vi "ex_BTD.vi"() -> ()   [LabVIEW 2022 SP3]
doc: "This is the VI which is a simple Blood Test Device"
uses:
  #typedef_Blood_Testing_Device_Task.ctl
  #typedef_Kind_Of_Operation_BTD.ctl
  #typedef_Blood_Testing_Device_States.ctl
  #typedef_TimerAction.ctl
  #typed_BTD_ProgramData.ctl
panel:
  out "Centrifugation (slide)":bool
  out "Kind Of Opeartion":T1
  in  "Lid Open":bool
  in  "Centrifugation":bool
  in  "Start":bool
  in  "Dial":T2 scale=0.0..4.0
  in  "stop":bool
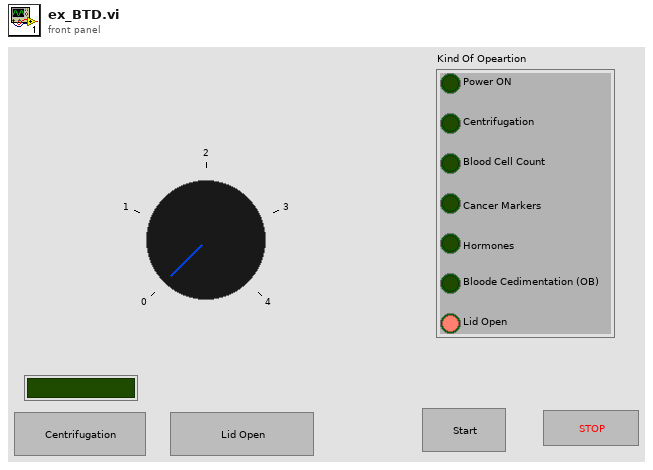
[diagram p1: front panel]
types:
  T1 = typedef "#typedef_Kind_Of_Operation_BTD.ctl" = cluster{"Power ON":bool, "Centrifugation":bool, "Blood Cell Count":bool, "Cancer Markers":bool, "Hormones":bool, "Bloode Cedimentation (OB)":bool, "Lid Open":bool}
  T2 = typedef "#typedef_Blood_Testing_Device_Task.ctl" = i32
  T3 = typedef "#typedef_Blood_Testing_Device_States.ctl" = enum16{"Blood Cedimentation (OB)", "Hormones", "Cancer Markers", "Blood Cell Count", "Centrifugation", "Initialization", "Exit", "Error Handler", "Centrifugation Led On", "Wait For Event"}
  T4 = typedef "#typedef_TimerAction.ctl" = enum16{"Reset", "TimeElapsed"}
  T5 = typedef "#typed_BTD_ProgramData.ctl" = cluster{"Kind Of Opearion":T1, "Task":T2}
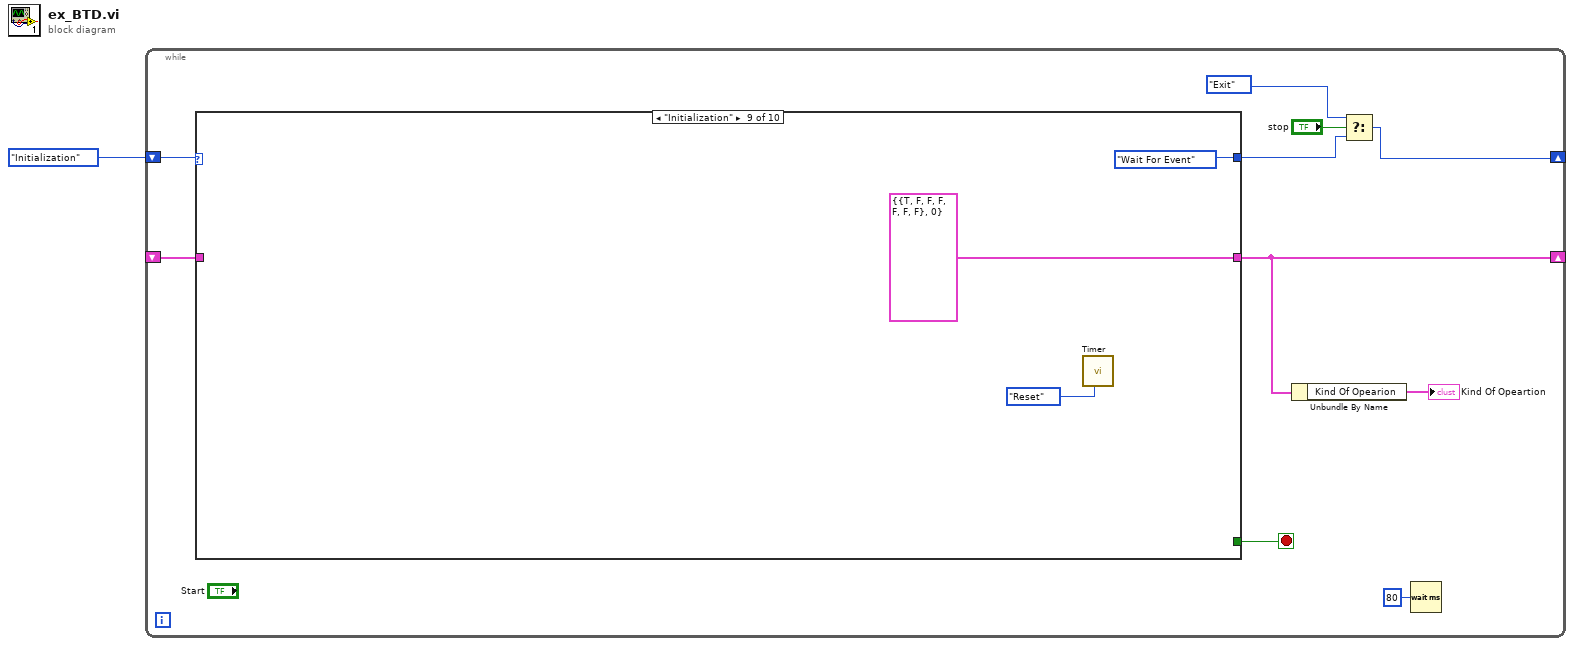
[diagram p0: block diagram]
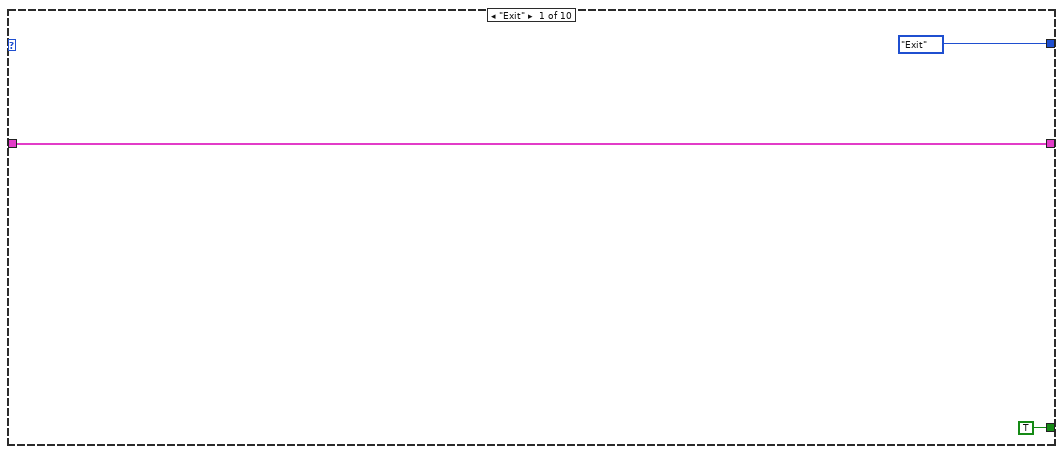
[diagram p2: hidden frame]
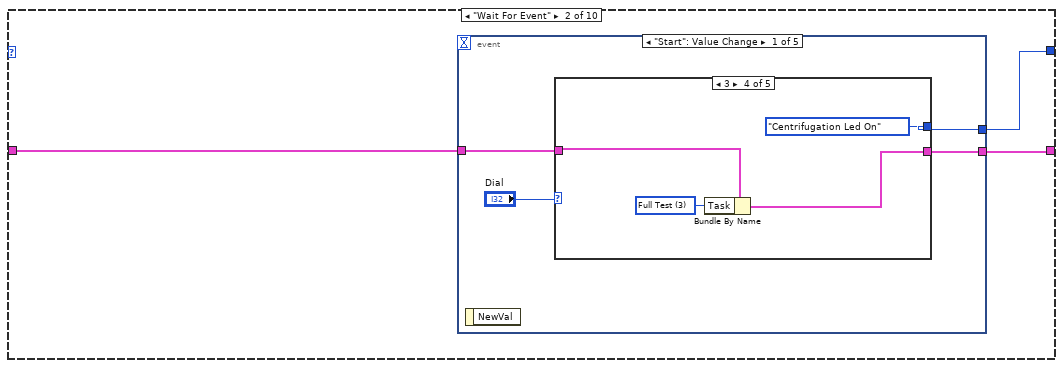
[diagram p3: hidden frame]
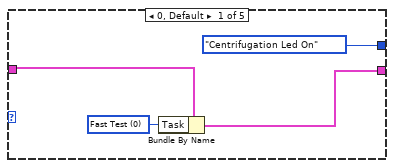
[diagram p4: hidden frame]
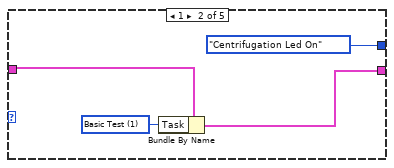
[diagram p5: hidden frame]
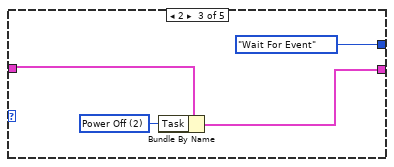
[diagram p6: hidden frame]
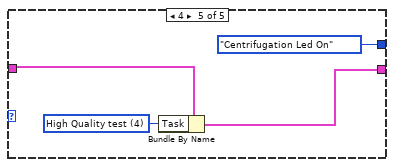
[diagram p7: hidden frame]
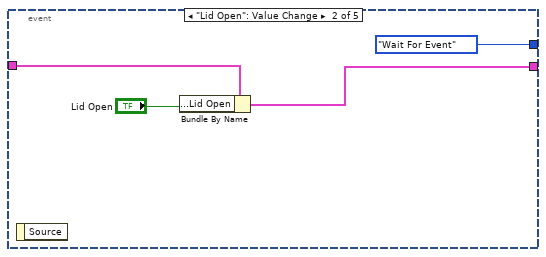
[diagram p8: hidden frame]
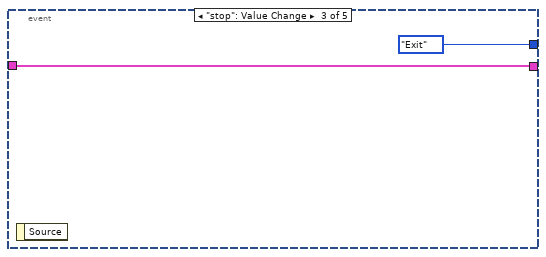
[diagram p9: hidden frame]
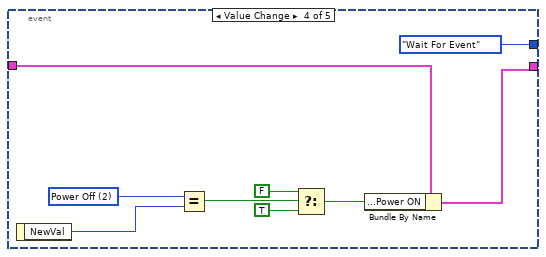
[diagram p10: hidden frame]
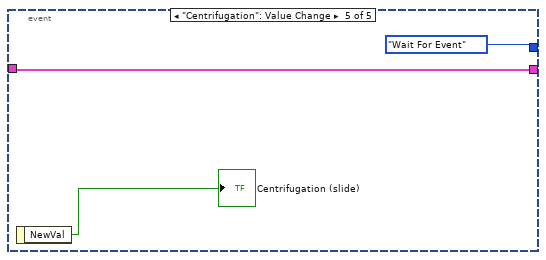
[diagram p11: hidden frame]
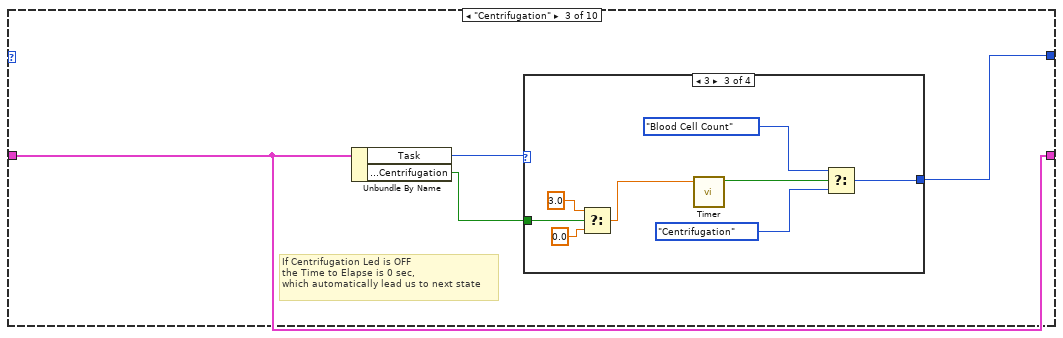
[diagram p12: hidden frame]
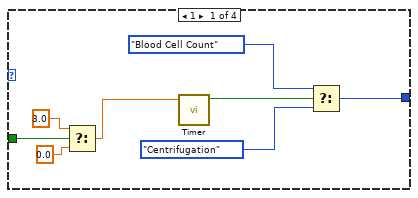
[diagram p13: hidden frame]
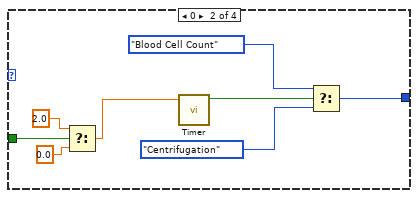
[diagram p14: hidden frame]
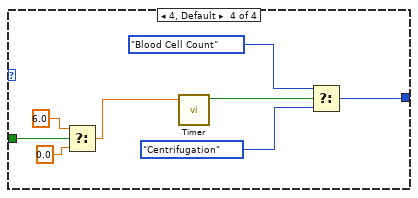
[diagram p15: hidden frame]
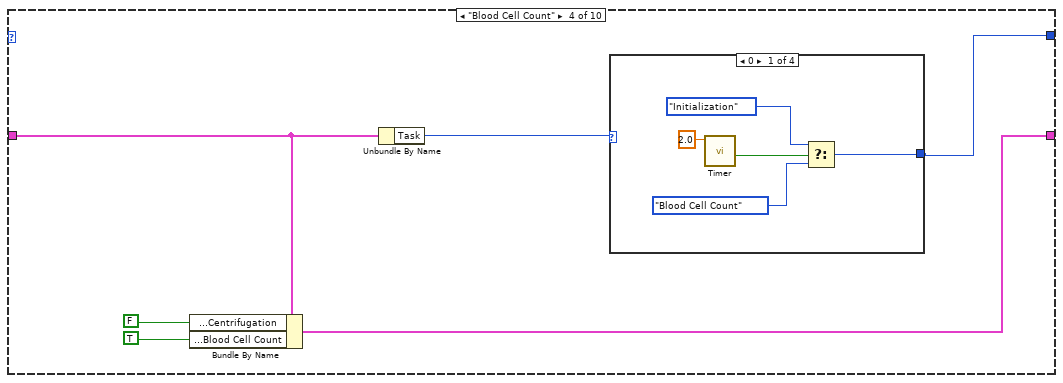
[diagram p16: hidden frame]
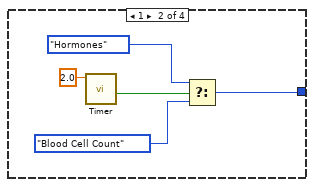
[diagram p17: hidden frame]
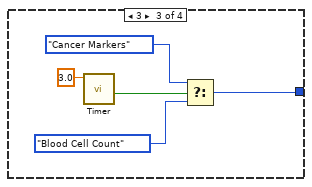
[diagram p18: hidden frame]
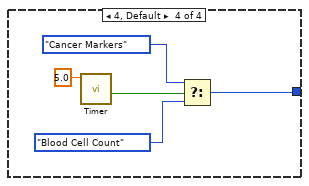
[diagram p19: hidden frame]
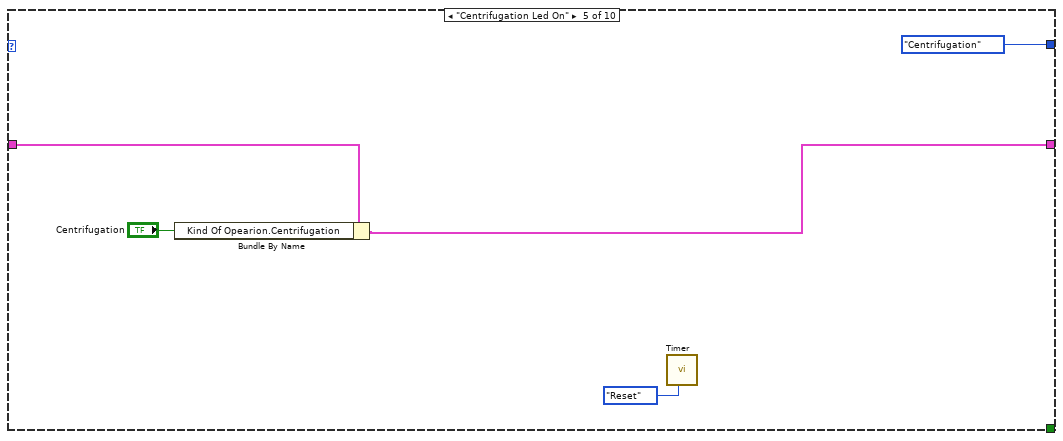
[diagram p20: hidden frame]
diagram:
  n1 = while {
    shift-right: [w4] -> _
    shift-left: #typedef_Blood_Testing_Device_States."Initialization" ("SM_States") -> [w11]
    shift-right: [w3] -> _
    shift-left: _ -> [w10]
    stop <- w9 stop-if-true
    n2 = case shown="\"Initialization\"" w11 {
      tunnel: [w13 w16 w60 w98 w124 w129 w146 w167 T5 {"Kind Of Opearion"={"Power ON"=TRUE, "Centrifugation"=FALSE, "Blood Cell Count"=FALSE, "Cancer Markers"=FALSE, "Hormones"=FALSE, "Bloode Cedimentation (OB)"=FALSE, "Lid Open"=FALSE}, "Task"=0} ("BTD_ProgramData") w190] -> w3
      tunnel: [#typedef_Blood_Testing_Device_States."Exit" ("SM_States") w15 w62 w97 #typedef_Blood_Testing_Device_States."Centrifugation" ("SM_States") w128 w145 w166 #typedef_Blood_Testing_Device_States."Wait For Event" ("SM_States") #typedef_Blood_Testing_Device_States."Exit" ("SM_States")] -> w7
      tunnel: w10 -> [w13 w17 w60 w100 w126 w131 w148 w169 _ w190]
      tunnel: [TRUE _ _ _ _ _ _ _ _ w189] -> w9
      frame "Exit" {
      }
      frame "Wait For Event" {
        n3 = event shown="[0] \"Start\": Value Change" {
          selector: _ -> [_ _ _ _ _]
          dyn-events: _ -> [_ _ _ _ _]
          timeout: _ -> [_ _ _ _ _]
          tunnel: w17 -> [w20 w45 w47 w50 w57]
          tunnel: [w19 w43 w47 w49 w57] -> w16
          tunnel: [w18 #typedef_Blood_Testing_Device_States."Wait For Event" ("SM_States") #typedef_Blood_Testing_Device_States."Exit" ("SM_States") #typedef_Blood_Testing_Device_States."Wait For Event" ("SM_States") #typedef_Blood_Testing_Device_States."Wait For Event" ("SM_States")] -> w15
          event "Start": Value Change {
            n4 = event-data() -> ()  [unwired: 1 in, 1 out]
            n5 = case shown="3" "Dial" {
              tunnel: w20 -> [w25 w29 w33 w37 w41]
              tunnel: [w23 w27 w31 w35 w39] -> w19
              tunnel: [#typedef_Blood_Testing_Device_States."Centrifugation Led On" ("SM_States") #typedef_Blood_Testing_Device_States."Centrifugation Led On" ("SM_States") #typedef_Blood_Testing_Device_States."Wait For Event" ("SM_States") #typedef_Blood_Testing_Device_States."Centrifugation Led On" ("SM_States") #typedef_Blood_Testing_Device_States."Centrifugation Led On" ("SM_States")] -> w18
              frame 0, Default {
                w24 = T2 0 items=["Fast Test", "Basic Test", "Power Off", "Full Test", "High Quality test"] ("Task")
                n6 = Bundle By Name(cluster=w25, "Task"=w24) -> (w23:T5)
              }
              frame 1 {
                w28 = T2 1 items=["Fast Test", "Basic Test", "Power Off", "Full Test", "High Quality test"] ("Task")
                n7 = Bundle By Name(cluster=w29, "Task"=w28) -> (w27:T5)
              }
              frame 2 {
                w32 = T2 2 items=["Fast Test", "Basic Test", "Power Off", "Full Test", "High Quality test"] ("Task")
                n8 = Bundle By Name(cluster=w33, "Task"=w32) -> (w31:T5)
              }
              frame 3 {
                w36 = T2 3 items=["Fast Test", "Basic Test", "Power Off", "Full Test", "High Quality test"] ("Task")
                n9 = Bundle By Name(cluster=w37, "Task"=w36) -> (w35:T5)
              }
              frame 4 {
                w40 = T2 4 items=["Fast Test", "Basic Test", "Power Off", "Full Test", "High Quality test"] ("Task")
                n10 = Bundle By Name(cluster=w41, "Task"=w40) -> (w39:T5)
              }
            }
          }
          event "Lid Open": Value Change {
            n11 = event-data() -> ()  [unwired: 1 in, 1 out]
            n12 = Bundle By Name(cluster=w45, "Kind Of Opearion.Lid Open"="Lid Open") -> (w43:T5)
          }
          event "stop": Value Change {
            n13 = event-data() -> ()  [unwired: 1 in, 1 out]
          }
          event Value Change {
            w52 = T2 2 items=["Fast Test", "Basic Test", "Power Off", "Full Test", "High Quality test"] ("x")
            n14 = event-data() -> ("NewVal"=w56:T2)  [unwired: 1 in]
            n15 = Equal?(x=w52, y=w56) -> (x = y?=w55:bool)
            n16 = Select(t=FALSE, s=w55, f=TRUE) -> (s? t:f=w51:bool)
            n17 = Bundle By Name(cluster=w50, "Kind Of Opearion.Power ON"=w51) -> (w49:T5)
          }
          event "Centrifugation": Value Change {
            n18 = event-data() -> ("NewVal"=→"Centrifugation (slide)":bool)  [unwired: 1 in]
          }
        }
      }
      frame "Centrifugation" {
        # "If Centrifugation Led is OFF\nthe Time to Elapse is 0 sec,\nwhich automatically lead us to next state"
        n19 = Unbundle By Name(w60) -> ("Task"=w63:T2, "Kind Of Opearion.Centrifugation"=w61:bool)
        n20 = case shown="3" w63 {
          tunnel: [w68 w76 w84 w92] -> w62
          tunnel: w61 -> [w67 w75 w83 w91]
          frame 1 {
            n21 = Select(t=3.0, s=w67, f=0.0) -> (s? t:f=w64:dbl)
            n22 = call "Timer.vi"("Time To Elapse"=w64) -> ("Time Elapsed?"=w70:bool)  [unwired: 8 in, 2 out]
            n23 = Select(t=#typedef_Blood_Testing_Device_States."Blood Cell Count" ("SM_States"), s=w70, f=#typedef_Blood_Testing_Device_States."Centrifugation") -> (s? t:f=w68:T3)
          }
          frame 0 {
            n24 = Select(t=2.0, s=w75, f=0.0) -> (s? t:f=w72:dbl)
            n25 = call "Timer.vi"("Time To Elapse"=w72) -> ("Time Elapsed?"=w78:bool)  [unwired: 8 in, 2 out]
            n26 = Select(t=#typedef_Blood_Testing_Device_States."Blood Cell Count" ("SM_States"), s=w78, f=#typedef_Blood_Testing_Device_States."Centrifugation") -> (s? t:f=w76:T3)
          }
          frame 3 {
            n27 = Select(t=3.0, s=w83, f=0.0) -> (s? t:f=w80:dbl)
            n28 = call "Timer.vi"("Time To Elapse"=w80) -> ("Time Elapsed?"=w86:bool)  [unwired: 8 in, 2 out]
            n29 = Select(t=#typedef_Blood_Testing_Device_States."Blood Cell Count" ("SM_States"), s=w86, f=#typedef_Blood_Testing_Device_States."Centrifugation") -> (s? t:f=w84:T3)
          }
          frame 4, Default {
            n30 = Select(t=6.0, s=w91, f=0.0) -> (s? t:f=w88:dbl)
            n31 = call "Timer.vi"("Time To Elapse"=w88) -> ("Time Elapsed?"=w94:bool)  [unwired: 8 in, 2 out]
            n32 = Select(t=#typedef_Blood_Testing_Device_States."Blood Cell Count" ("SM_States"), s=w94, f=#typedef_Blood_Testing_Device_States."Centrifugation") -> (s? t:f=w92:T3)
          }
        }
      }
      frame "Blood Cell Count" {
        n33 = Bundle By Name(cluster=w100, "Kind Of Opearion.Centrifugation"=FALSE, "Kind Of Opearion.Blood Cell Count"=TRUE) -> (w98:T5)
        n34 = Unbundle By Name(w100) -> ("Task"=w101:T2)
        n35 = case shown="0" w101 {
          tunnel: [w102 w107 w112 w117] -> w97
          frame 0 {
            n36 = call "Timer.vi"("Time To Elapse"=2.0) -> ("Time Elapsed?"=w106:bool)  [unwired: 8 in, 2 out]
            n37 = Select(t=#typedef_Blood_Testing_Device_States."Initialization" ("SM_States"), s=w106, f=#typedef_Blood_Testing_Device_States."Blood Cell Count" ("SM_States")) -> (s? t:f=w102:T3)
          }
          frame 1 {
            n38 = call "Timer.vi"("Time To Elapse"=2.0) -> ("Time Elapsed?"=w111:bool)  [unwired: 8 in, 2 out]
            n39 = Select(t=#typedef_Blood_Testing_Device_States."Hormones" ("SM_States"), s=w111, f=#typedef_Blood_Testing_Device_States."Blood Cell Count" ("SM_States")) -> (s? t:f=w107:T3)
          }
          frame 3 {
            n40 = call "Timer.vi"("Time To Elapse"=3.0) -> ("Time Elapsed?"=w116:bool)  [unwired: 8 in, 2 out]
            n41 = Select(t=#typedef_Blood_Testing_Device_States."Cancer Markers" ("SM_States"), s=w116, f=#typedef_Blood_Testing_Device_States."Blood Cell Count" ("SM_States")) -> (s? t:f=w112:T3)
          }
          frame 4, Default {
            n42 = call "Timer.vi"("Time To Elapse"=5.0) -> ("Time Elapsed?"=w121:bool)  [unwired: 8 in, 2 out]
            n43 = Select(t=#typedef_Blood_Testing_Device_States."Cancer Markers" ("SM_States"), s=w121, f=#typedef_Blood_Testing_Device_States."Blood Cell Count" ("SM_States")) -> (s? t:f=w117:T3)
          }
        }
      }
      frame "Centrifugation Led On" {
        n44 = Bundle By Name(cluster=w126, "Kind Of Opearion.Centrifugation"="Centrifugation") -> (w124:T5)
        n45 = call "Timer.vi"("Action (Time Elapsed)"=#typedef_TimerAction."Reset") -> ()  [unwired: 8 in, 3 out]
      }
      frame "Cancer Markers" {
        n46 = Bundle By Name(cluster=w131, "Kind Of Opearion.Blood Cell Count"=FALSE ("Kind Of Opearion.Centrifugation"), "Kind Of Opearion.Cancer Markers"=TRUE ("Kind Of Opearion.Blood Cell Count")) -> (w129:T5)
        n47 = Unbundle By Name(w131) -> ("Task"=w132:T2)
        n48 = case shown="4, Default" w132 {
          tunnel: [w133 w138] -> w128
          frame 3 {
            n49 = call "Timer.vi"("Time To Elapse"=3.0) -> ("Time Elapsed?"=w137:bool)  [unwired: 8 in, 2 out]
            n50 = Select(t=#typedef_Blood_Testing_Device_States."Hormones" ("SM_States"), s=w137, f=#typedef_Blood_Testing_Device_States."Cancer Markers" ("SM_States")) -> (s? t:f=w133:T3)
          }
          frame 4, Default {
            n51 = call "Timer.vi"("Time To Elapse"=6.0) -> ("Time Elapsed?"=w142:bool)  [unwired: 8 in, 2 out]
            n52 = Select(t=#typedef_Blood_Testing_Device_States."Hormones" ("SM_States"), s=w142, f=#typedef_Blood_Testing_Device_States."Cancer Markers" ("SM_States")) -> (s? t:f=w138:T3)
          }
        }
      }
      frame "Hormones" {
        n53 = Bundle By Name(cluster=w148, "Kind Of Opearion.Blood Cell Count"=FALSE, "Kind Of Opearion.Cancer Markers"=FALSE ("Kind Of Opearion.Centrifugation"), "Kind Of Opearion.Hormones"=TRUE ("Kind Of Opearion.Blood Cell Count")) -> (w146:T5)
        n54 = Unbundle By Name(w148) -> ("Task"=w149:T2)
        n55 = case shown="1, Default" w149 {
          tunnel: [w150 w155 w160] -> w145
          frame 3 {
            n56 = call "Timer.vi"("Time To Elapse"=3.0) -> ("Time Elapsed?"=w154:bool)  [unwired: 8 in, 2 out]
            n57 = Select(t=#typedef_Blood_Testing_Device_States."Blood Cedimentation (OB)" ("SM_States"), s=w154, f=#typedef_Blood_Testing_Device_States."Hormones" ("SM_States")) -> (s? t:f=w150:T3)
          }
          frame 4 {
            n58 = call "Timer.vi"("Time To Elapse"=5.0) -> ("Time Elapsed?"=w159:bool)  [unwired: 8 in, 2 out]
            n59 = Select(t=#typedef_Blood_Testing_Device_States."Blood Cedimentation (OB)" ("SM_States"), s=w159, f=#typedef_Blood_Testing_Device_States."Hormones" ("SM_States")) -> (s? t:f=w155:T3)
          }
          frame 1, Default {
            n60 = call "Timer.vi"("Time To Elapse"=3.0) -> ("Time Elapsed?"=w164:bool)  [unwired: 8 in, 2 out]
            n61 = Select(t=#typedef_Blood_Testing_Device_States."Blood Cedimentation (OB)" ("SM_States"), s=w164, f=#typedef_Blood_Testing_Device_States."Hormones" ("SM_States")) -> (s? t:f=w160:T3)
          }
        }
      }
      frame "Blood Cedimentation (OB)" {
        n62 = Bundle By Name(cluster=w169, "Kind Of Opearion.Hormones"=FALSE ("Kind Of Opearion.Centrifugation"), "Kind Of Opearion.Bloode Cedimentation (OB)"=TRUE ("Kind Of Opearion.Blood Cell Count")) -> (w167:T5)
        n63 = Unbundle By Name(w169) -> ("Task"=w170:T2)
        n64 = case shown="4, Default" w170 {
          tunnel: [w171 w176 w181] -> w166
          frame 3 {
            n65 = call "Timer.vi"("Time To Elapse"=3.0) -> ("Time Elapsed?"=w175:bool)  [unwired: 8 in, 2 out]
            n66 = Select(t=#typedef_Blood_Testing_Device_States."Initialization" ("SM_States"), s=w175, f=#typedef_Blood_Testing_Device_States."Blood Cedimentation (OB)" ("SM_States")) -> (s? t:f=w171:T3)
          }
          frame 4, Default {
            n67 = call "Timer.vi"("Time To Elapse"=6.0) -> ("Time Elapsed?"=w180:bool)  [unwired: 8 in, 2 out]
            n68 = Select(t=#typedef_Blood_Testing_Device_States."Initialization" ("SM_States"), s=w180, f=#typedef_Blood_Testing_Device_States."Blood Cedimentation (OB)" ("SM_States")) -> (s? t:f=w176:T3)
          }
          frame 1 {
            n69 = call "Timer.vi"("Time To Elapse"=2.0) -> ("Time Elapsed?"=w185:bool)  [unwired: 8 in, 2 out]
            n70 = Select(t=#typedef_Blood_Testing_Device_States."Initialization" ("SM_States"), s=w185, f=#typedef_Blood_Testing_Device_States."Blood Cedimentation (OB)" ("SM_States")) -> (s? t:f=w181:T3)
          }
        }
      }
      frame "Initialization" {
        n71 = call "Timer.vi"("Action (Time Elapsed)"=#typedef_TimerAction."Reset") -> ()  [unwired: 8 in, 3 out]
      }
      frame "Error Handler" {
        n72 = One Button Dialog(message="Application Error!") -> (true=w189:bool)  [unwired: 1 in]
      }
    }
    n73 = Unbundle By Name(w3) -> ("Kind Of Opearion"=→"Kind Of Opeartion":T1)
    n74 = Select(t=#typedef_Blood_Testing_Device_States."Exit" ("SM_States"), s="stop", f=w7) -> (s? t:f=w4:T3)
    n75 = Wait (ms)(milliseconds to wait=u32 80) -> ()  [unwired: 1 out]
  }
